vi "Framework_Initialize.vi"(8 "error in (no error)":errorcluster, 11 "Class in":refnum<class "Installer.lvclass">) -> (0 "error out":errorcluster, 1 "helpTopics":string[](array[string]), 2 "pageTitles":string[](array[string]), 3 "Class out":refnum<class "Installer.lvclass">, 4 "helpFile":string, 5 "pages":path[](array[path]))   [LabVIEW 2020, in "Installer.lvclass"]
uses:
  <vilib>/AppBuilder/IB_Classes/Installer/Installer.lvclass
  <vilib>/AppBuilder/IB_Classes/Installer/Installer.lvclass/Installer.ctl
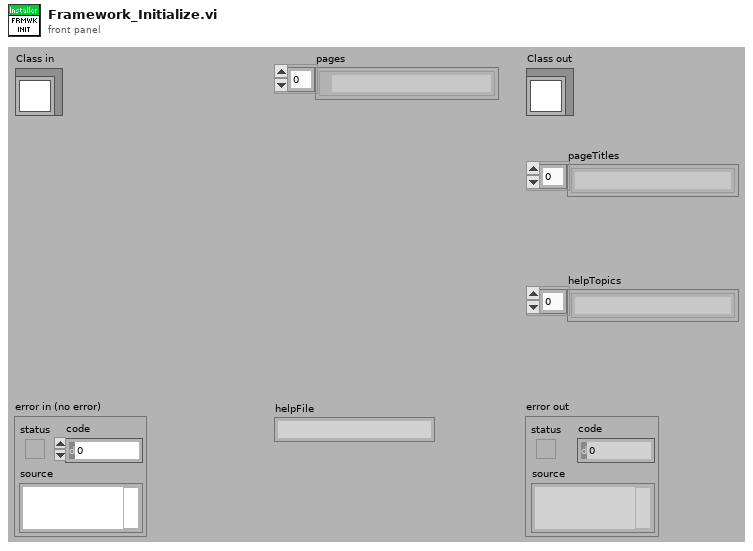
[diagram p1: front panel]
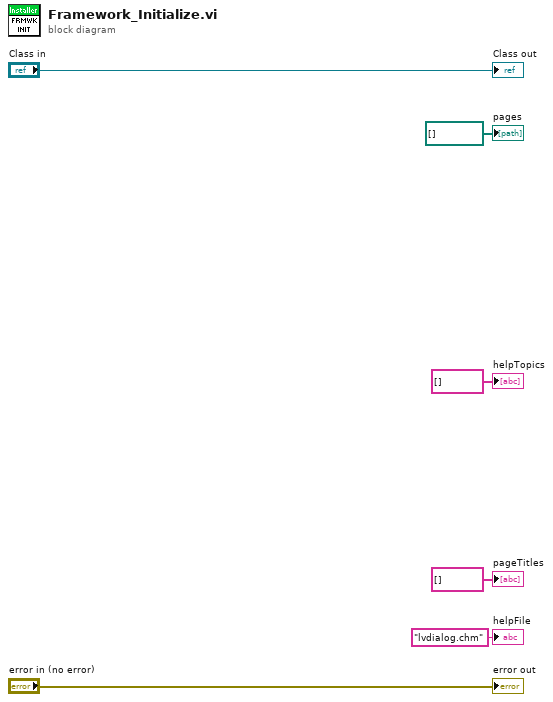
[diagram p0: block diagram]
diagram:
  "error out" <- "error in (no error)"
  "Class out" <- "Class in"
  "pages" <- path[] [] ("pages")
  "helpTopics" <- string[] [] ("helpTopics")
  "pageTitles" <- string[] [] ("pageTitles")
  "helpFile" <- "lvdialog.chm" ("helpFile")
